vi "ble_cmd_connection_disconnect.vi"(6 "Connection Status":T1={"MAC Address"="", "cnx handle"=0, "cnx flags"=0, "Address Type"=125, "Connection Interval (ms)"=125, "Timeout(ms)"=125, "Latency"=0, "bonding handle"=0} {"Address Type" items=["Public", "Random"]}, 8 "error in (no error)":errorcluster, 11 "COM Bluegiga in":refnum<visa-resource-name>) -> (0 "error out":errorcluster, 3 "COM Bluegiga out":refnum<visa-resource-name>)   [LabVIEW 2015]
uses:
  type_def/connection_status_bundle.ctl
  type_def/address_type.ctl
  type_def/message_class.ctl
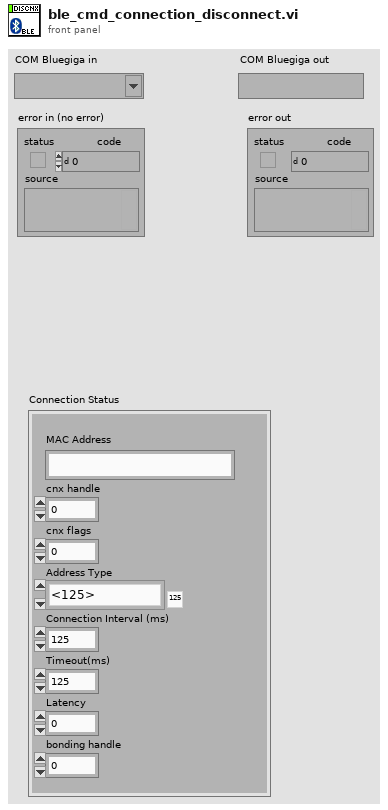
[diagram p1: front panel]
types:
  T1 = typedef "connection_status_bundle.ctl" = cluster{"MAC Address":string, "cnx handle":u8, "cnx flags":u8, "Address Type":T2, "Connection Interval (ms)":u16, "Timeout(ms)":u16, "Latency":u16, "bonding handle":u8}
  T2 = typedef "address_type.ctl" = u8
  T3 = typedef "message_class.ctl" = u8
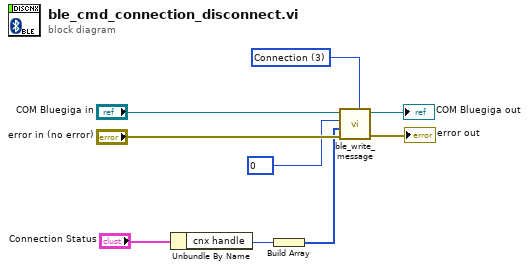
[diagram p0: block diagram]
diagram:
  w3 = T3 3 items=["System", "Persistent Store", "Attribute database", "Connection", "Attribute client", "Security Manager", "Generic Access Profile", "Hardware"] ("Command Class (System)")
  n1 = Unbundle By Name("Connection Status") -> ("cnx handle"=w5:u8)
  n2 = Build Array(w5) -> (w4:u8[])
  n3 = call "ble_write_message.vi"("Command Class (System)"=w3, "error in (no error)"="error in (no error)", "Payload(Empty)"=w4, "Message ID (0x00)"=u8 0, "COM Bluegiga in"="COM Bluegiga in") -> ("error out"=→"error out":errorcluster, "COM Bluegiga out"=→"COM Bluegiga out":refnum<visa-resource-name>)  [unwired: 4 in, 1 out]
